vi "Write Gain Selection.vi"(8 "error in (no error)":errorcluster, 10 "Gain Values":T1 items=["+/-6.144V (2/3)"=0, "+/-4.096V (1)"=512, "+/-2.048V (2)"=1024, "+/-1.024V (4)"=1536, "+/-0.512V (8)"=2048, "+/-0.256V (16)"=2560], 11 "LINX-ADS1X15 in":refnum<class "LINX-ADS1X15.lvclass">) -> (0 "error out":errorcluster, 3 "LINX-ADS1X15 out":refnum<class "LINX-ADS1X15.lvclass">)   [LabVIEW 2020, in "LINX-ADS1X15.lvclass"]
uses:
  LINX-ADS1X15.lvclass
  Programmable Gain Selection.ctl
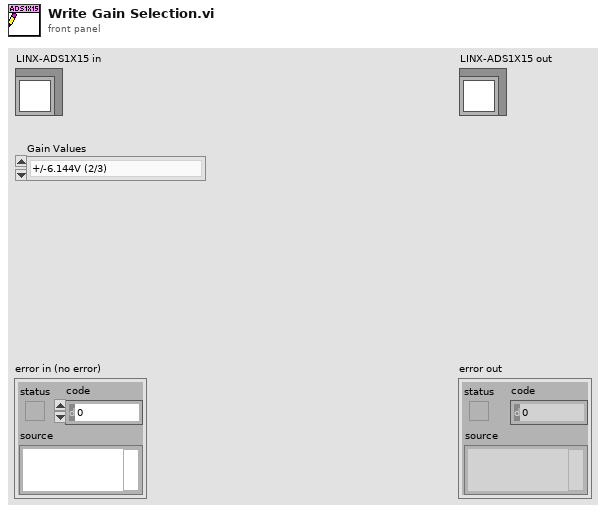
[diagram p1: front panel]
types:
  T1 = typedef "LINX-ADS1X15.lvclass/Programmable Gain Selection.ctl" = u16
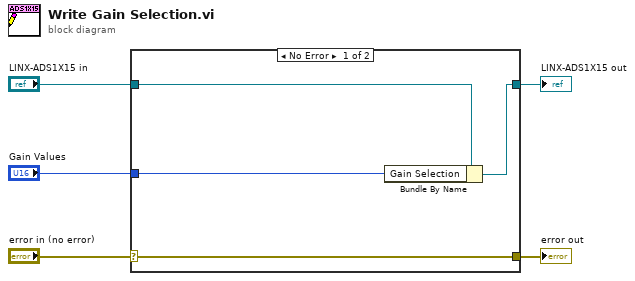
[diagram p0: block diagram]
diagram:
  n1 = case shown="No Error" "error in (no error)" {
    selector: "error in (no error)" -> [w9 w10]
    tunnel: [w9 w10] -> w4
    tunnel: [w7 w11] -> w2
    tunnel: "LINX-ADS1X15 in" -> [w8 w11]
    tunnel: "Gain Values" -> [w6 _]
    frame No Error {
      n2 = Bundle By Name(cluster=w8, "Gain Selection"=w6) -> (w7:refnum<class "LINX-ADS1X15.lvclass">)
    }
    frame Error {
    }
  }
  "error out" <- w4
  "LINX-ADS1X15 out" <- w2
